vi "LJUD_GoOne.vi"(8 "error in":errorcluster, 11 "Handle In":i32) -> (0 "error out":errorcluster, 3 "Handle Out":i32)   [LabVIEW 2021]
doc: "GoOne executes a list of requests\non a single device.\n\nThis is a traditional technique UD\nfunction ... Add-Add-Go-Get-Get.\nSee Section 4.1 of the device's\ndatasheet for more information.."
uses:
  labjackud.dll
panel:
  # "GoOne executes a list of requests\non a single device.\n\nThis is a traditional technique UD\nfunction ... Add-Add-Go-Get-Get.\nSee Section 4.1 of the device's\ndatasheet for more information.."
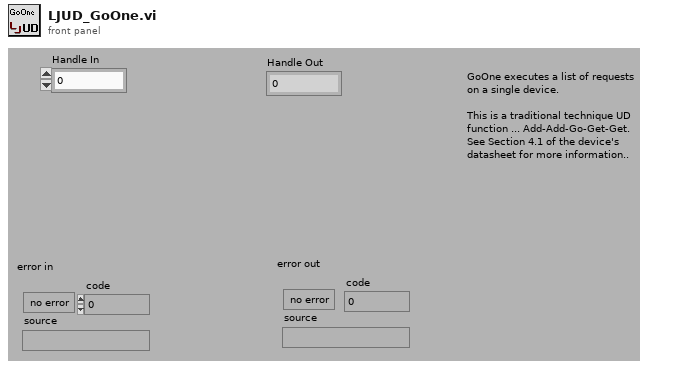
[diagram p1: front panel]
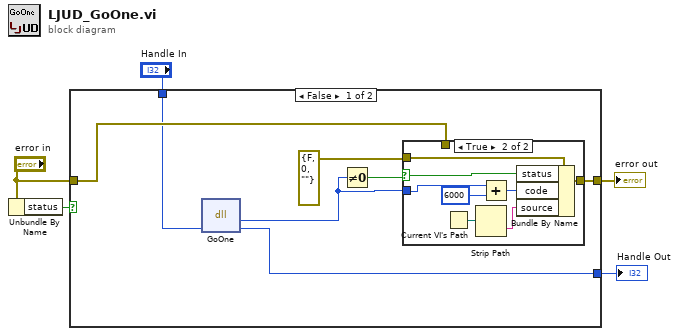
[diagram p0: block diagram]
diagram:
  n1 = Unbundle By Name("error in") -> ("status"=w4:bool)
  n2 = case shown="False" w4 {
    tunnel: [w10 w23] -> w5
    tunnel: "error in" -> [w8 w23]
    tunnel: "Handle In" -> [w7 w22]
    tunnel: [w6 w22] -> w1
    frame False {
      n3 = dll-call lib="labjackud.dll" fn="GoOne"("Handle"=w7) -> (w11:i32, "Handle"=w6:i32)  [unwired: 3 in, 2 out]
      n4 = Not Equal To 0?(x=w11) -> (x != 0?=w9:bool)
      n5 = case shown="True" w9 {
        selector: w9 -> [_ w20]
        tunnel: [w13 w21] -> w10
        tunnel: errorcluster {"status"=FALSE, "code"=0, "source"=""} ("error IO") -> [_ w19]
        tunnel: w11 -> [_ w15]
        tunnel: w8 -> [w13 _]
        frame False {
        }
        frame True {
          n6 = Current VI's Path() -> (path=w17:path)
          n7 = Strip Path(path=w17) -> (name=w18:string)  [unwired: 1 out]
          n8 = Add(x=w15, y=6000) -> (x+y=w16:i32)
          n9 = Bundle By Name(cluster=w19, "status"=w20, "code"=w16, "source"=w18) -> (w21:errorcluster)
        }
      }
    }
    frame True {
    }
  }
  "error out" <- w5
  "Handle Out" <- w1
